vi "insertElement.vi"(8 "error in (no error)":errorcluster, 9 "index":i32=-1, 10 "ScriptEvent":refnum<class "ScriptEvent.lvclass">, 11 "ScriptEventList in":refnum<class "ScriptEventList.lvclass">) -> (0 "error out":errorcluster, 3 "ScriptEventList out":refnum<class "ScriptEventList.lvclass">)   [LabVIEW 2009, in "Tools.lvlib" / "Scripting.lvlib" / "ScriptEventList.lvclass"]
uses:
  ScriptEventList.lvclass
  ScriptEvent.lvclass
  ScriptEventList.lvclass/ScriptEventList.ctl
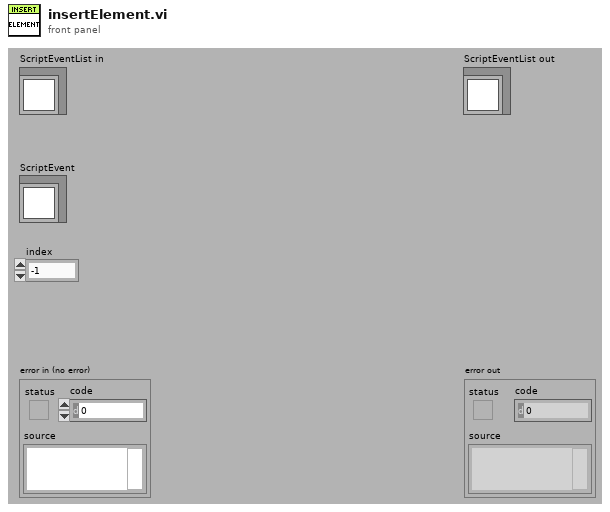
[diagram p1: front panel]
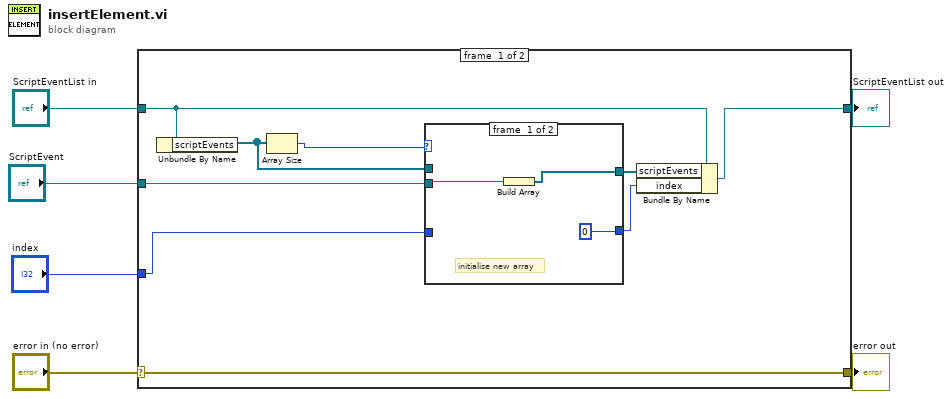
[diagram p0: block diagram]
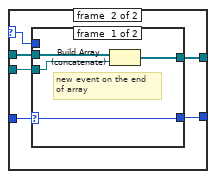
[diagram p2: hidden frame]
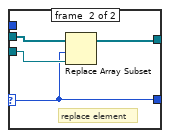
[diagram p3: hidden frame]
diagram:
  n1 = case shown="No Error" "error in (no error)" {
    selector: "error in (no error)" -> [w15 w34]
    tunnel: [w15 w34] -> w5
    tunnel: [w8 w33] -> w3
    tunnel: "ScriptEventList in" -> [w9 w33]
    tunnel: "ScriptEvent" -> [w11 _]
    tunnel: "index" -> [w12 _]
    frame #0 {
      n2 = Unbundle By Name(w9) -> ("scriptEvents"=w13:refnum<class "ScriptEvent.lvclass">[])
      n3 = Array Size(array=w13) -> (size(s)=w14:i32)
      n4 = case shown="Default" w14 {
        selector: w14 -> [_ w20]
        tunnel: w13 -> [_ w24]
        tunnel: w12 -> [_ w23]
        tunnel: w11 -> [w18 w22]
        tunnel: [w17 w21] -> w10
        tunnel: [0 w19] -> w7
        frame #0 {
          # "initialise new array"
          n5 = Build Array(w18) -> (w17:refnum<class "ScriptEvent.lvclass">[])
        }
        frame #1 {
          n6 = case shown="-1" w23 {
            selector: w23 -> [w25 w29]
            tunnel: w24 -> [w28 w32]
            tunnel: w22 -> [w27 w31]
            tunnel: [w26 w30] -> w21
            tunnel: w20 -> [_ _]
            tunnel: [w25 w29] -> w19
            frame #0 {
              # "new event on the end\nof array"
              n7 = Build Array (concatenate)(w28, w27) -> (w26:refnum<class "ScriptEvent.lvclass">[])
            }
            frame #1 {
              # "replace element"
              n8 = Replace Array Subset(array=w32, new element=w31, index=w29) -> (w30:refnum<class "ScriptEvent.lvclass">[])
            }
          }
        }
      }
      n9 = Bundle By Name(cluster=w9, "scriptEvents"=w10, "index"=w7) -> (w8:refnum<class "ScriptEventList.lvclass">)
    }
    frame #1 {
    }
  }
  "error out" <- w5
  "ScriptEventList out" <- w3
